vi "VisualizeNetwork.vi"() -> ()   [LabVIEW 2014, in "Visualization.lvlib" / "VisualizeNetwork_class.lvclass"]
uses:
  VisualizeNetwork_class.lvclass
  Framework/Bus_class/Bus.lvclass
  VisializeBase_class/Typedefs/VisualizeData.ctl
  VisializeBase_class/Typedefs/clVisualizeData.ctl
  Modules/EventPlugins/EventPluginBaseClass/TypeDefs/clEvtReportArray.ctl
  Modules/EventPlugins/EventPluginBaseClass/TypeDefs/clEvtReport.ctl
  Modules/EventPlugins/EventPluginBaseClass/TypeDefs/dblEvtSignalArray.ctl
  Modules/NetworkImpairmentModule/PublicAPI/Arguments/Broadcasts/dblNetworkTime.ctl
  Modules/NetworkImpairmentModule/PublicAPI/Arguments/Broadcasts/dblPktLoss.ctl
  Modules/FlagImpairModule/PublicAPI/Arguments/Broadcasts/ui32FlagImpairmentArray.ctl
  Framework/Bus_class/Broadcast/Typedefs/clDidInit.ctl
  QMH/Typedefs/clNetImpairmentTime.ctl
  QMH/Typedefs/clNetIPktLoss.ctl
  QMH/Typedefs/clFlagImpairArray.ctl
  VisializeBase_class/Requests/clUserEventType.ctl
  <vilib>/event_ctls.llb/usereventprio.ctl
  <vilib>/Utility/miscctls.llb/LVStringsAndValuesArrayTypeDef_U8.ctl
  QMH/Typedefs/clEvtRptArray.ctl
  QMH/Typedefs/clPmuImpairRptArray.ctl
  QMH/Typedefs/clEvtRptSignal.ctl
  <vilib>/Utility/error.llb/Error Cluster From Error Code.vi
  <vilib>/ErrorRing/Error Ring.xnode
  VisializeBase_class/VisualizeBase_class.lvclass
  <userlib>/NIST/NISTErrorLib/NISTErrorLib.lvlib
  Framework/Bus_class/Bus_class.lvlib
  Modules/EventModule/EventModule.lvlib
  Modules/PmuImpairModule/PmuImpairModule.lvlib
  Modules/NetworkImpairmentModule/NetworkImpairmentModule.lvlib
  Modules/FlagImpairModule/FlagImpairModule.lvlib
  Modules/EventPlugins/EventPluginBaseClass/EventPluginBaseClass.lvclass
  VisualizeApp_class/VisualizeAppBase_class.lvclass
panel:
  in  "QueName":string="NetQue"
  out "ImpairPlot":cluster{dbl[], i32[]}[](graph) caption="Event Outputs and Impaired Network Outputs Over Time"
  out "Total Network Delay":T1(graph)
  out "Lost Packets":cluster{"NetworkTime":dbl, "BusIndex":u16}[](graph)
  in  "Bus Number":u8(ring) items=["", "1"]
  out "ErrorArray":errorcluster[](array[cluster])
  in  "btnStop":bool
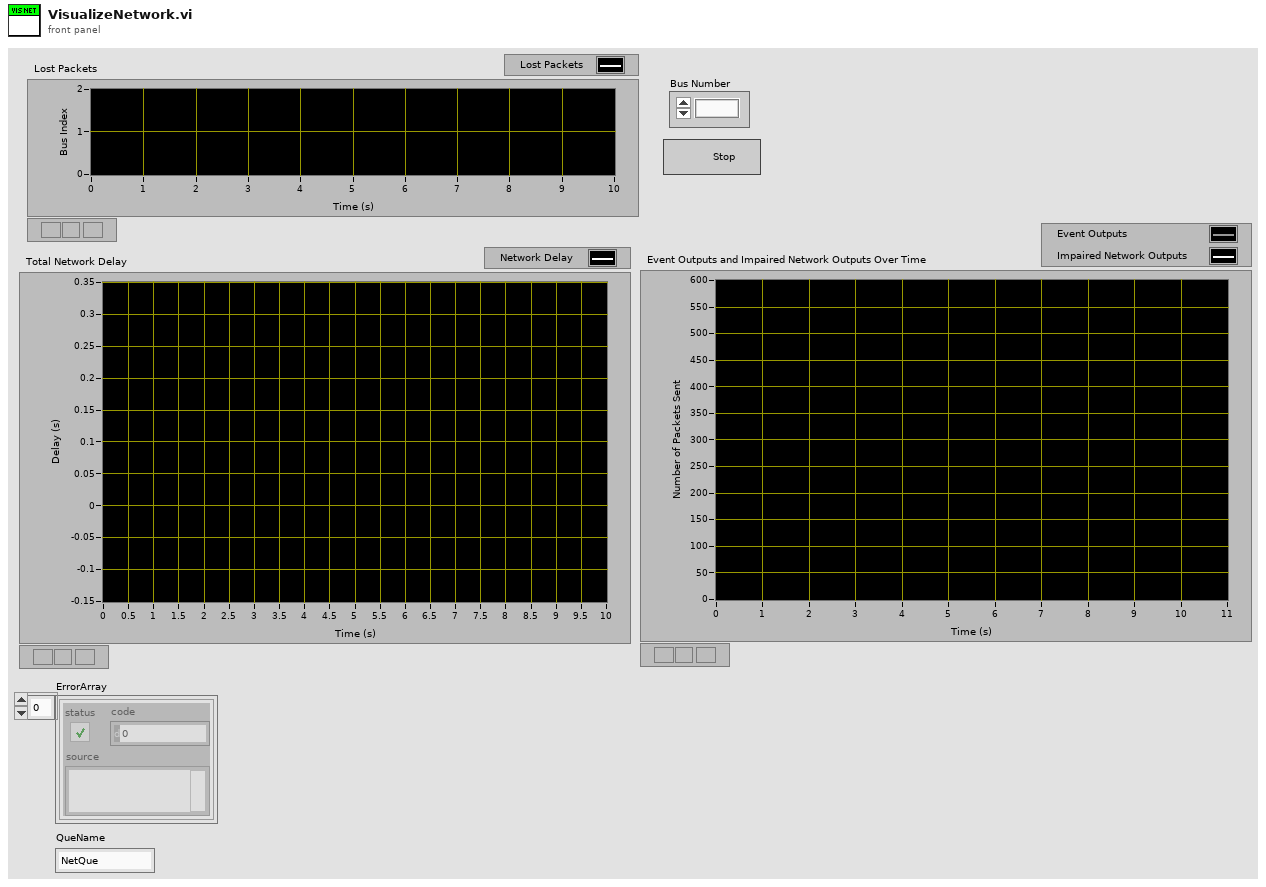
[diagram p1: front panel]
types:
  T1 = cluster{"dblNetworkTime":dbl[], "TimeArray":dbl[]}
  T2 = typedef "Visualization.lvlib/VisualizeBase_class.lvclass/VisualizeData.ctl" = T3[]
  T3 = typedef "Visualization.lvlib/VisualizeAppBase_class.lvclass/clVisualizeData.ctl" = cluster{"clEvtReportArray":T4, "dblEventSignalArray":T6, "clPmuImpairRptArray":T4, "dblNetworkTime":T7, "dblPktLoss":T8, "FlagImpairArray":T9, "TimeArray":dbl[]}
  T4 = typedef "EventPlugins.lvlib/EventPluginBaseClass.lvclass/clEvtReportArray.ctl" = T5[]
  T5 = typedef "EventPlugins.lvlib/EventPluginBaseClass.lvclass/clEvtReport.ctl" = cluster{"Timestamp":dbl, "Synx":cdb[], "Freq":dbl, "ROCOF":dbl, "ID":i16}
  T6 = typedef "EventPlugins.lvlib/EventPluginBaseClass.lvclass/dblEvtSignalArray.ctl" = dbl[][]
  T7 = typedef "NetworkImpairmentModule.lvlib/dblNetworkTime.ctl" = dbl[]
  T8 = typedef "NetworkImpairmentModule.lvlib/dblPktLoss.ctl" = dbl[]
  T9 = typedef "FlagImpairModule.lvlib/ui32FlagImpairmentArray.ctl" = u32[]
  T10 = typedef "Visualization.lvlib/VisualizeBase_class.lvclass/clRequestEvents.ctl" = cluster{"StopRequest":refnum<user-event>}
  T11 = typedef "Bus_class.lvlib/clBroadcastEvents.ctl" = cluster{"DidInit":refnum<user-event>, "DidStop":refnum<user-event>}
  T12 = typedef "EventModule.lvlib/clBroadcastEvents.ctl" = cluster{"DidInit":refnum<user-event>, "StatusUpdate":refnum<user-event>, "ErrorReport":refnum<user-event>, "DidStop":refnum<user-event>, "ReadEvtConfig":refnum<user-event>, "ReadTimeArray":refnum<user-event>, "ReadEvtParams":refnum<user-event>, "GetEvtReportArray":refnum<user-event>, "ReadPathToPlugin":refnum<user-event>, "GetEvtSignal":refnum<user-event>, "ReadBusNumber":refnum<user-event>}
  T13 = typedef "PmuImpairModule.lvlib/clBroadcastEvents.ctl" = cluster{"DidInit":refnum<user-event>, "StatusUpdate":refnum<user-event>, "ErrorReport":refnum<user-event>, "DidStop":refnum<user-event>, "ImpairConfig":refnum<user-event>, "ImpairParams":refnum<user-event>, "ImpairReports":refnum<user-event>, "PathToPlugin":refnum<user-event>, "BusNumber":refnum<user-event>}
  T14 = typedef "NetworkImpairmentModule.lvlib/clBroadcastEvents.ctl" = cluster{"DidInit":refnum<user-event>, "StatusUpdate":refnum<user-event>, "ErrorReport":refnum<user-event>, "DidStop":refnum<user-event>, "ReadNetImpParams":refnum<user-event>, "ReadLossThreshold":refnum<user-event>, "GetNetworkTime":refnum<user-event>, "GetPktLoss":refnum<user-event>, "ReadPathToPlugin":refnum<user-event>}
  T15 = typedef "FlagImpairModule.lvlib/clBroadcastEvents.ctl" = cluster{"DidInit":refnum<user-event>, "StatusUpdate":refnum<user-event>, "ErrorReport":refnum<user-event>, "DidStop":refnum<user-event>, "ReadFlagImpairConfig":refnum<user-event>, "ReadPluginINIFilePath":refnum<user-event>, "ReadFlagImpairParams":refnum<user-event>, "ReadTimeArray":refnum<user-event>, "GetFlagImpairment":refnum<user-event>}
  T16 = cluster{"BusNumberRef":refnum<vi>, "ImpairPlot":refnum<vi>, "Lost Packets":refnum<vi>, "Total Network Delay":refnum<vi>}
  T17 = typedef "LVStringsAndValuesArrayTypeDef_U8.ctl" = cluster{"String":string, "Value":u8}[]
  T18 = typedef "Visualization.lvlib/VisualizeBase_class.lvclass/clEvtRptArray.ctl" = cluster{"BusIndex":i32, "clImpairReportArray":T4}
  T19 = typedef "Visualization.lvlib/VisualizeBase_class.lvclass/clPmuImpairRptArray.ctl" = cluster{"BusIndex":i32, "clImpairReportArray":T4}
  T20 = typedef "Visualization.lvlib/VisualizeBase_class.lvclass/clNetImpairmentTime.ctl" = cluster{"BusIndex":i32, "clNetImpairTimeArray":T7}
  T21 = typedef "Visualization.lvlib/VisualizeBase_class.lvclass/clNetIPktLoss.ctl" = cluster{"BusIndex":i32, "clNetPktLoss":T8}
  T22 = typedef "Visualization.lvlib/VisualizeBase_class.lvclass/clFlagImpairArray.ctl" = cluster{"BusIndex":i32, "FlagImpairArray":T9}
  T23 = typedef "Visualization.lvlib/VisualizeBase_class.lvclass/clEvtRptSignal.ctl" = cluster{"BusIndex":i32, "dblEventSignalArray":T6}
  T24 = typedef "Visualization.lvlib/VisualizeBase_class.lvclass/clUserEventType.ctl" = cluster{"BusIndex":i8, "Data":variant}
  T25 = typedef "usereventprio.ctl" = enum32{"high priority", "normal priority"}
  T26 = typedef "Bus_class.lvlib/clDidInit.ctl" = cluster{"Bus":refnum<vi>, "Init?":bool}
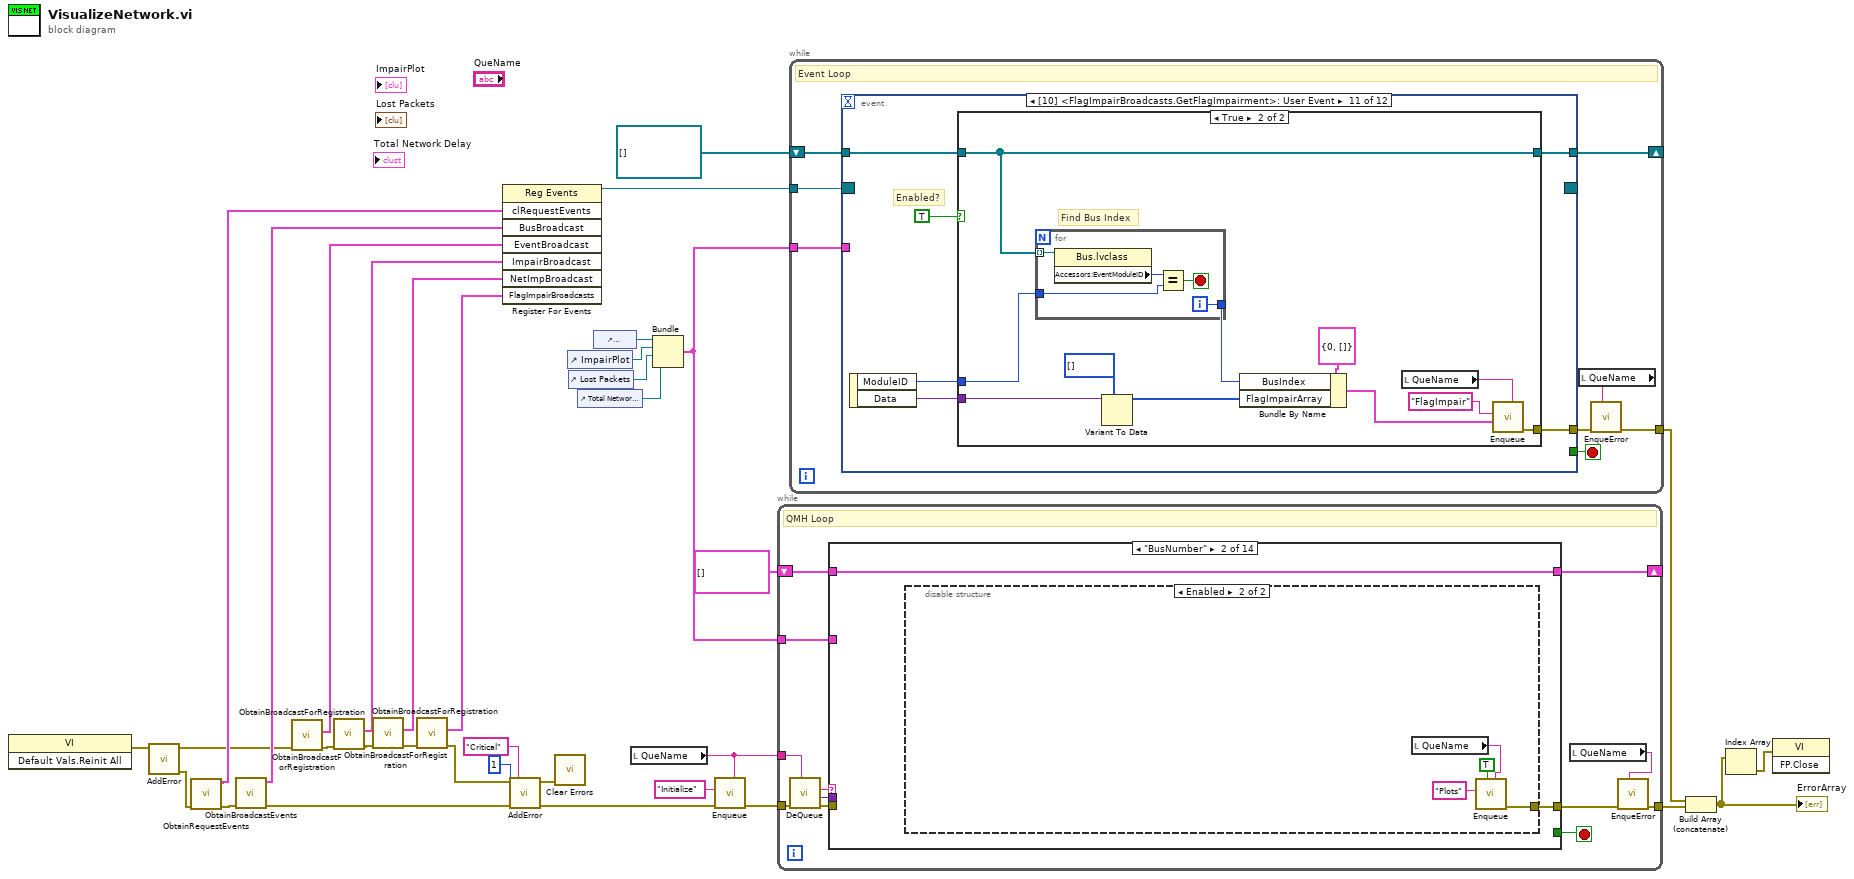
[diagram p0: block diagram]
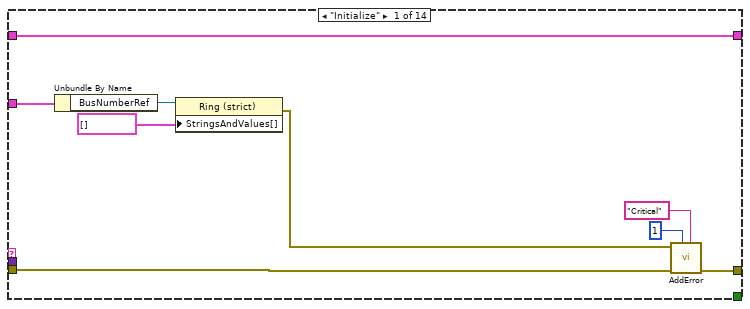
[diagram p2: hidden frame]
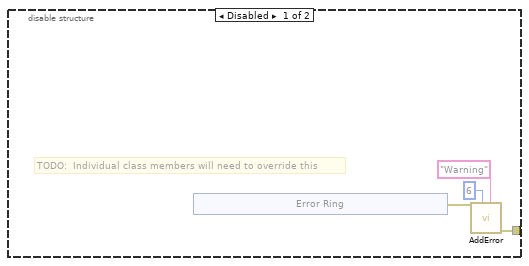
[diagram p3: hidden frame]
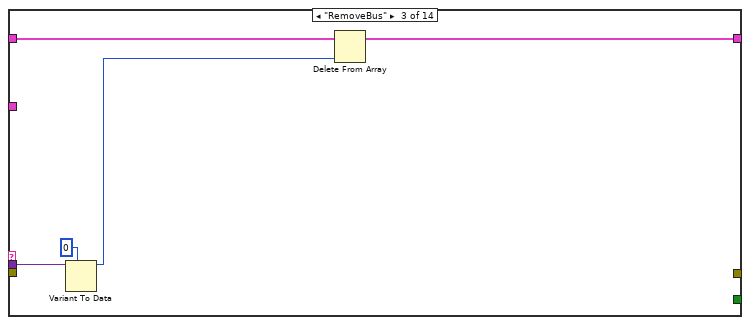
[diagram p4: hidden frame]
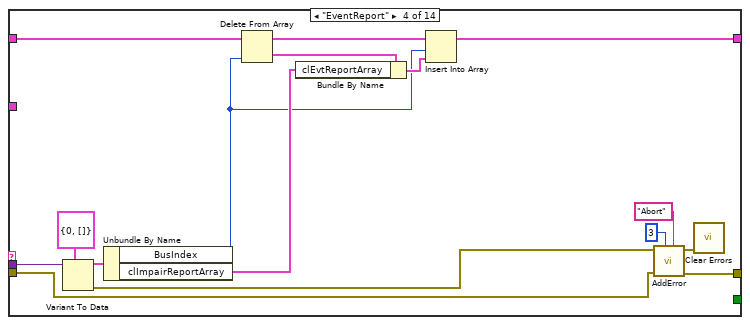
[diagram p5: hidden frame]
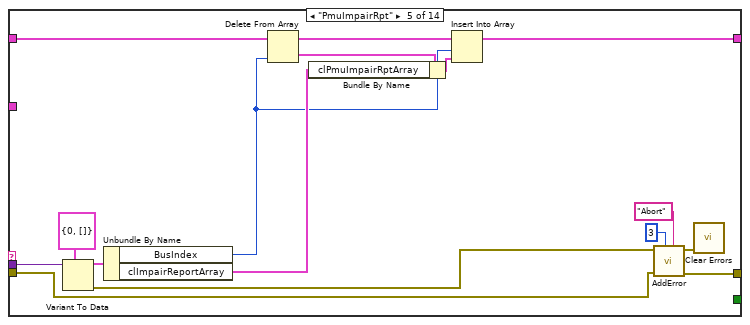
[diagram p6: hidden frame]
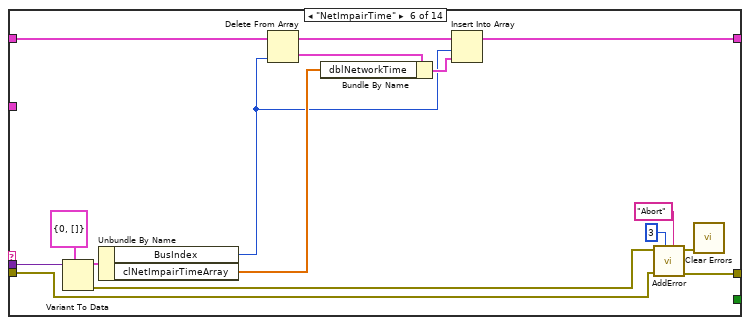
[diagram p7: hidden frame]
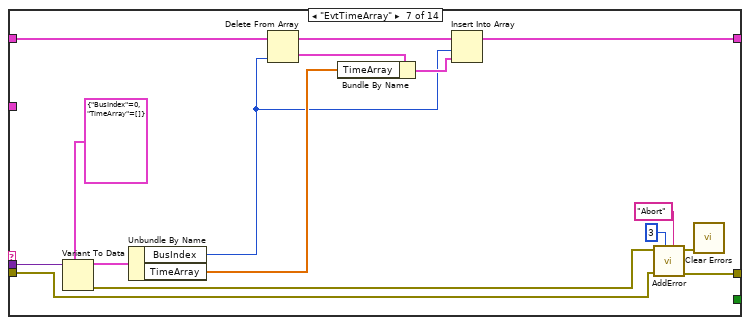
[diagram p8: hidden frame]
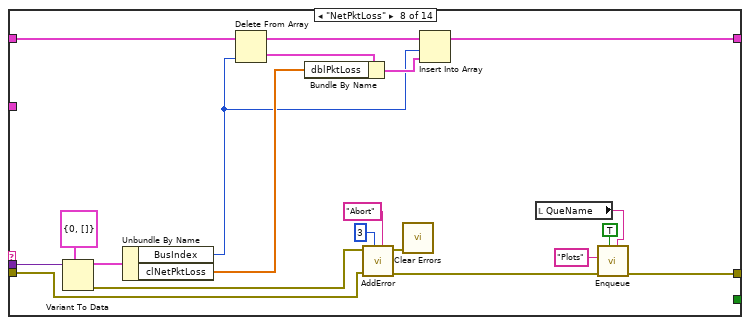
[diagram p9: hidden frame]
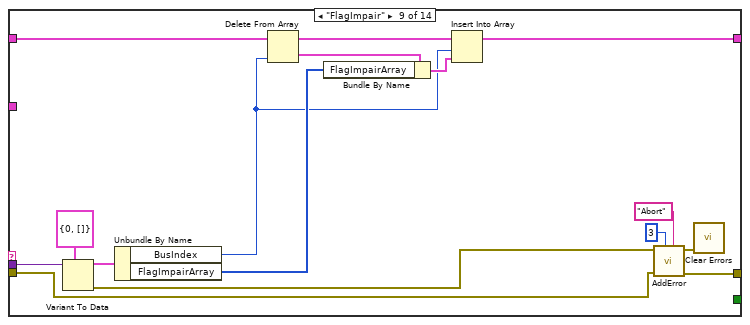
[diagram p10: hidden frame]
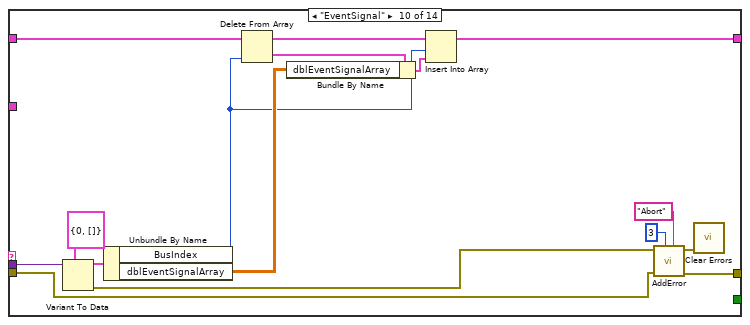
[diagram p11: hidden frame]
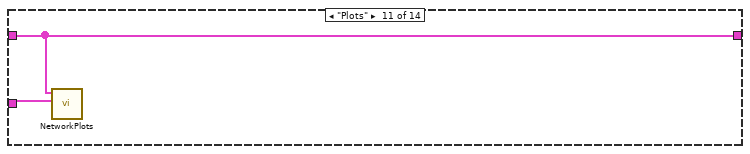
[diagram p12: hidden frame]
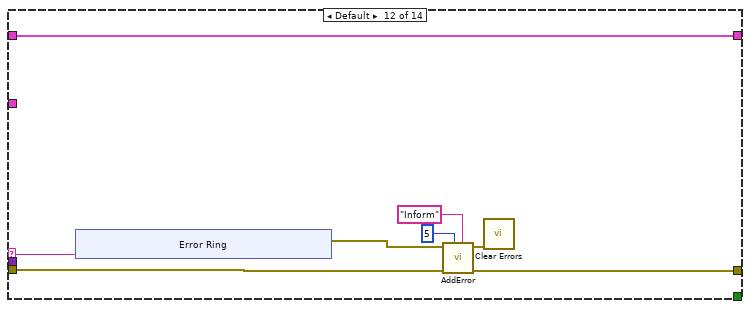
[diagram p13: hidden frame]
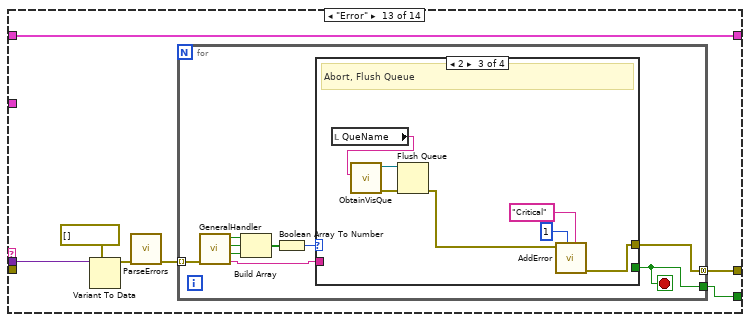
[diagram p14: hidden frame]
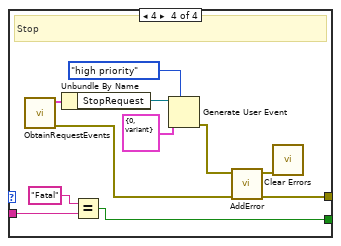
[diagram p17: hidden frame]
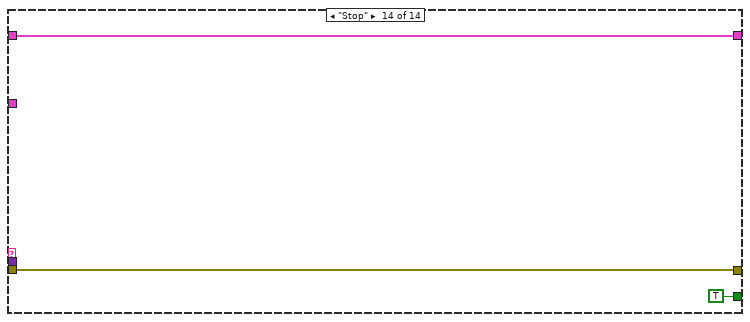
[diagram p18: hidden frame]
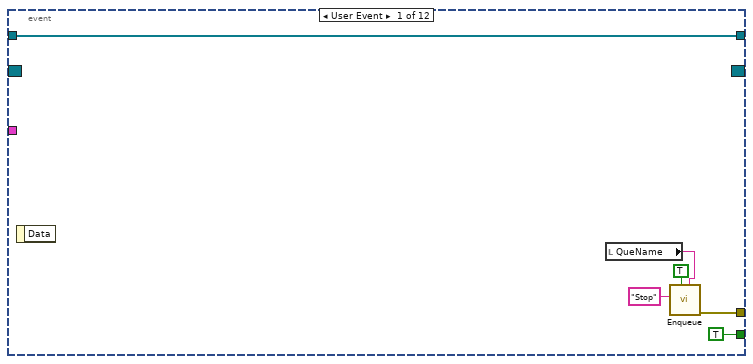
[diagram p19: hidden frame]
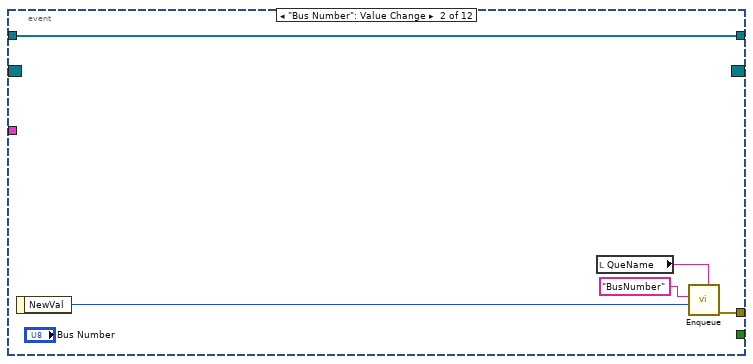
[diagram p20: hidden frame]
diagram:
  n1 = invoke class="VI" method="Default Vals.Reinit All"() -> (error out=w24:errorcluster)  [unwired: 3 in, 2 out]
  n2 = call <userlib>:"AddError.vi"("error in (no error)"=w24) -> ("ErrorArray"=w23:errorcluster[], "error out"=w15:errorcluster)  [unwired: 9 in]
  n3 = call "ObtainRequestEvents.vi"("Error"=w23) -> ("Error"=w28:errorcluster[], "clRequestEvents"=w32:T10)  [unwired: 9 in]
  n4 = call "ObtainBroadcastEvents.vi"("ErrorArray"=w28) -> ("ErrorArray"=w14:errorcluster[], "BusBroadcast"=w27:T11)  [unwired: 9 in]
  n5 = call "ObtainBroadcastForRegistration.vi"("error in (no error)"=w15) -> ("error out"=w18:errorcluster, "EventBroadcast"=w22:T12)  [unwired: 9 in]
  n6 = call "ObtainBroadcastForRegistration.vi"("error in (no error)"=w18) -> ("error out"=w17:errorcluster, "ImpairBroadcast"=w21:T13)  [unwired: 9 in]
  n7 = call "ObtainBroadcastForRegistration.vi"("error in (no error)"=w17) -> ("error out"=w16:errorcluster, "NetImpBroadcast"=w20:T14)  [unwired: 9 in]
  n8 = call "ObtainBroadcastForRegistration.vi"("error in (no error)"=w16) -> ("error out"=w13:errorcluster, "FlagImpairBroadcasts"=w19:T15)  [unwired: 9 in]
  n9 = register-events(w32, w27, w22, w21, w20, w19) -> (reference out=w31:refnum<event-registration>)  [unwired: 2 in, 1 out]
  n10 = call <userlib>:"AddError.vi"("Severity"="Critical" ("String"), "Priority"=u8 1, "ErrorArray"=w14, "error in (no error)"=w13) -> ("ErrorArray"=w10:errorcluster[], "error out"=w7:errorcluster)  [unwired: 6 in]
  n11 = call <vilib>:"Clear Errors.vi"("error in (no error)"=w7) -> ()  [unwired: 5 in, 2 out]
  n12 = control-ref of="ImpairPlot"() -> (w4:refnum<vi>)
  n13 = control-ref of="Lost Packets"() -> (w6:refnum<vi>)
  n14 = control-ref of="Total Network Delay"() -> (w5:refnum<vi>)
  n15 = control-ref of="BusNumberRef"() -> (w26:refnum<vi>)
  n16 = local read "QueName"() -> (w3:string)
  n17 = Bundle("BusNumberRef"=w26, "ImpairPlot"=w4, "Lost Packets"=w6, "Total Network Delay"=w5) -> (w8:T16)  [unwired: 1 in]
  n18 = call "Enqueue.vi"("QueName"=w3, "Error"=w10, "Message"="Initialize") -> ("Error"=w33:errorcluster[])  [unwired: 8 in]
  n19 = while {
    tunnel: w33 -> [w46]
    tunnel: [w40] -> w30
    tunnel: w8 -> [w39]
    shift-right: [w37] -> _
    shift-left: T2 [] ("VisualizeData") -> [w38]
    tunnel: w3 -> [w36]
    stop <- w41 stop-if-true
    # "QMH Loop"
    n20 = call "DeQueue.vi"("QueName"=w36, "Error"=w46) -> ("Error"=w43:errorcluster[], "Data"=w44:variant, "Message"=w45:string)  [unwired: 7 in]
    n21 = case shown="\"BusNumber\"" w45 {
      selector: w45 -> [_ _ _ _ _ _ _ _ _ _ _ w201 _ _]
      tunnel: w44 -> [_ _ w75 w91 w107 w123 w139 w159 w175 w191 _ _ w215 _]
      tunnel: w43 -> [w52 _ _ w76 w92 w108 w125 w145 w160 w176 _ w199 _ w244]
      tunnel: [w51 w57 _ w81 w97 w113 w130 w143 w165 w181 _ w198 w211 w244] -> w42
      tunnel: [_ _ _ _ _ _ _ _ _ _ _ _ w210 TRUE] -> w41
      tunnel: w39 -> [w55 _ _ _ _ _ _ _ _ _ w192 _ _ _]
      tunnel: w38 -> [w47 w56 w73 w87 w103 w119 w136 w155 w171 w187 w193 w194 w209 w243]
      tunnel: [w47 w56 w72 w88 w104 w120 w137 w156 w172 w188 w193 w194 w209 w243] -> w37
      frame "Initialize" {
        n22 = Unbundle By Name(w55) -> ("BusNumberRef"=w54:refnum<vi>)
        n23 = property class="Ring (strict)"(reference=w54, "StringsAndValues[]"=T17 [] ("Strings And Values []")) -> (error out=w50:errorcluster)  [unwired: 1 in, 1 out]
        n24 = call <userlib>:"AddError.vi"("Severity"="Critical" ("String"), "Priority"=u8 1, "ErrorArray"=w52, "error in (no error)"=w50) -> ("ErrorArray"=w51:errorcluster[])  [unwired: 6 in, 1 out]
      }
      frame "BusNumber" {
        n25 = disable-structure shown="Enabled" {
          disable-tunnel: [w61 w67] -> w57
          frame Disabled {
            # "TODO:  Individual class members will need to override this"
            n26 = xnode "Error Ring"() -> ("error out"=w60:errorcluster)
            n27 = call <userlib>:"AddError.vi"("Severity"="Warning" ("String"), "Priority"=u8 6, "error in (no error)"=w60) -> ("ErrorArray"=w61:errorcluster[])  [unwired: 7 in, 1 out]
          }
          frame Enabled {
            n28 = local read "QueName"() -> (w70:string)
            n29 = call "Enqueue.vi"("QueName"=w70, "Priority? (F)"=TRUE, "Message"="Plots") -> ("Error"=w67:errorcluster[])  [unwired: 8 in]
          }
        }
      }
      frame "RemoveBus" {
        n30 = Variant To Data(type=0, Variant=w75) -> (data=w71:i32)  [unwired: 1 in, 1 out]
        n31 = Delete From Array(array=w73, index=w71) -> (array with subset deleted=w72:T2)  [unwired: 1 in, 1 out]
      }
      frame "EventReport" {
        n32 = Variant To Data(type=T18 {"BusIndex"=0, "clImpairReportArray"=[]} ("clEvtReportArray"), Variant=w91) -> (data=w89:T18, error out=w80:errorcluster)  [unwired: 1 in]
        n33 = Unbundle By Name(w89) -> ("BusIndex"=w82:i32, "clImpairReportArray"=w84:T4)
        n34 = Delete From Array(array=w87, index=w82) -> (deleted portion=w85:T3, array with subset deleted=w86:T2)  [unwired: 1 in]
        n35 = Bundle By Name(cluster=w85, "clEvtReportArray"=w84) -> (w83:T3)
        n36 = Insert Into Array(array=w86, index=w82, new element=w83) -> (w88:T2)
        n37 = call <userlib>:"AddError.vi"("Severity"="Abort" ("String"), "Priority"=u8 3, "ErrorArray"=w76, "error in (no error)"=w80) -> ("ErrorArray"=w81:errorcluster[], "error out"=w79:errorcluster)  [unwired: 6 in]
        n38 = call <vilib>:"Clear Errors.vi"("error in (no error)"=w79) -> ()  [unwired: 5 in, 2 out]
      }
      frame "PmuImpairRpt" {
        n39 = Variant To Data(type=T19 {"BusIndex"=0, "clImpairReportArray"=[]} ("clImpairReportArray"), Variant=w107) -> (data=w105:T19, error out=w96:errorcluster)  [unwired: 1 in]
        n40 = Unbundle By Name(w105) -> ("BusIndex"=w98:i32, "clImpairReportArray"=w100:T4)
        n41 = Delete From Array(array=w103, index=w98) -> (deleted portion=w101:T3, array with subset deleted=w102:T2)  [unwired: 1 in]
        n42 = Bundle By Name(cluster=w101, "clPmuImpairRptArray"=w100) -> (w99:T3)
        n43 = Insert Into Array(array=w102, index=w98, new element=w99) -> (w104:T2)
        n44 = call <userlib>:"AddError.vi"("Severity"="Abort" ("String"), "Priority"=u8 3, "ErrorArray"=w92, "error in (no error)"=w96) -> ("ErrorArray"=w97:errorcluster[], "error out"=w95:errorcluster)  [unwired: 6 in]
        n45 = call <vilib>:"Clear Errors.vi"("error in (no error)"=w95) -> ()  [unwired: 5 in, 2 out]
      }
      frame "NetImpairTime" {
        n46 = Variant To Data(type=T20 {"BusIndex"=0, "clNetImpairTimeArray"=[]} ("clImpairReportArray"), Variant=w123) -> (data=w121:T20, error out=w112:errorcluster)  [unwired: 1 in]
        n47 = Unbundle By Name(w121) -> ("BusIndex"=w114:i32, "clNetImpairTimeArray"=w116:T7)
        n48 = Delete From Array(array=w119, index=w114) -> (deleted portion=w117:T3, array with subset deleted=w118:T2)  [unwired: 1 in]
        n49 = Bundle By Name(cluster=w117, "dblNetworkTime"=w116) -> (w115:T3)
        n50 = Insert Into Array(array=w118, index=w114, new element=w115) -> (w120:T2)
        n51 = call <userlib>:"AddError.vi"("Severity"="Abort" ("String"), "Priority"=u8 3, "ErrorArray"=w108, "error in (no error)"=w112) -> ("ErrorArray"=w113:errorcluster[], "error out"=w111:errorcluster)  [unwired: 6 in]
        n52 = call <vilib>:"Clear Errors.vi"("error in (no error)"=w111) -> ()  [unwired: 5 in, 2 out]
      }
      frame "EvtTimeArray" {
        n53 = Variant To Data(type=cluster{"BusIndex":i32, "TimeArray":dbl[]} {"BusIndex"=0, "TimeArray"=[]} ("cluster"), Variant=w139) -> (data=w138:cluster{"BusIndex":i32, "TimeArray":dbl[]}, error out=w129:errorcluster)  [unwired: 1 in]
        n54 = Unbundle By Name(w138) -> ("BusIndex"=w131:i32, "TimeArray"=w133:dbl[])
        n55 = Delete From Array(array=w136, index=w131) -> (deleted portion=w134:T3, array with subset deleted=w135:T2)  [unwired: 1 in]
        n56 = Bundle By Name(cluster=w134, "TimeArray"=w133) -> (w132:T3)
        n57 = Insert Into Array(array=w135, index=w131, new element=w132) -> (w137:T2)
        n58 = call <userlib>:"AddError.vi"("Severity"="Abort" ("String"), "Priority"=u8 3, "ErrorArray"=w125, "error in (no error)"=w129) -> ("ErrorArray"=w130:errorcluster[], "error out"=w128:errorcluster)  [unwired: 6 in]
        n59 = call <vilib>:"Clear Errors.vi"("error in (no error)"=w128) -> ()  [unwired: 5 in, 2 out]
      }
      frame "NetPktLoss" {
        n60 = Variant To Data(type=T21 {"BusIndex"=0, "clNetPktLoss"=[]} ("clNetPktLoss"), Variant=w159) -> (data=w157:T21, error out=w149:errorcluster)  [unwired: 1 in]
        n61 = Unbundle By Name(w157) -> ("BusIndex"=w150:i32, "clNetPktLoss"=w152:T8)
        n62 = Delete From Array(array=w155, index=w150) -> (deleted portion=w153:T3, array with subset deleted=w154:T2)  [unwired: 1 in]
        n63 = Bundle By Name(cluster=w153, "dblPktLoss"=w152) -> (w151:T3)
        n64 = call <userlib>:"AddError.vi"("Severity"="Abort" ("String"), "Priority"=u8 3, "ErrorArray"=w145, "error in (no error)"=w149) -> ("ErrorArray"=w144:errorcluster[], "error out"=w148:errorcluster)  [unwired: 6 in]
        n65 = call <vilib>:"Clear Errors.vi"("error in (no error)"=w148) -> ()  [unwired: 5 in, 2 out]
        n66 = Insert Into Array(array=w154, index=w150, new element=w151) -> (w156:T2)
        n67 = local read "QueName"() -> (w140:string)
        n68 = call "Enqueue.vi"("QueName"=w140, "Priority? (F)"=TRUE, "Error"=w144, "Message"="Plots") -> ("Error"=w143:errorcluster[])  [unwired: 7 in]
      }
      frame "FlagImpair" {
        n69 = Variant To Data(type=T22 {"BusIndex"=0, "FlagImpairArray"=[]} ("clFlagImpairArray"), Variant=w175) -> (data=w173:T22, error out=w164:errorcluster)  [unwired: 1 in]
        n70 = Unbundle By Name(w173) -> ("BusIndex"=w166:i32, "FlagImpairArray"=w168:T9)
        n71 = Delete From Array(array=w171, index=w166) -> (deleted portion=w169:T3, array with subset deleted=w170:T2)  [unwired: 1 in]
        n72 = Bundle By Name(cluster=w169, "FlagImpairArray"=w168) -> (w167:T3)
        n73 = Insert Into Array(array=w170, index=w166, new element=w167) -> (w172:T2)
        n74 = call <userlib>:"AddError.vi"("Severity"="Abort" ("String"), "Priority"=u8 3, "ErrorArray"=w160, "error in (no error)"=w164) -> ("ErrorArray"=w165:errorcluster[], "error out"=w163:errorcluster)  [unwired: 6 in]
        n75 = call <vilib>:"Clear Errors.vi"("error in (no error)"=w163) -> ()  [unwired: 5 in, 2 out]
      }
      frame "EventSignal" {
        n76 = Variant To Data(type=T23 {"BusIndex"=0, "dblEventSignalArray"=[]} ("clEvtReportArray"), Variant=w191) -> (data=w189:T23, error out=w180:errorcluster)  [unwired: 1 in]
        n77 = Unbundle By Name(w189) -> ("BusIndex"=w182:i32, "dblEventSignalArray"=w184:T6)
        n78 = Delete From Array(array=w187, index=w182) -> (deleted portion=w185:T3, array with subset deleted=w186:T2)  [unwired: 1 in]
        n79 = Bundle By Name(cluster=w185, "dblEventSignalArray"=w184) -> (w183:T3)
        n80 = Insert Into Array(array=w186, index=w182, new element=w183) -> (w188:T2)
        n81 = call <userlib>:"AddError.vi"("Severity"="Abort" ("String"), "Priority"=u8 3, "ErrorArray"=w176, "error in (no error)"=w180) -> ("ErrorArray"=w181:errorcluster[], "error out"=w179:errorcluster)  [unwired: 6 in]
        n82 = call <vilib>:"Clear Errors.vi"("error in (no error)"=w179) -> ()  [unwired: 5 in, 2 out]
      }
      frame "Plots" {
        n83 = call "NetworkPlots.vi"("ControlRefs"=w192, "VisualizeData"=w193) -> ()  [unwired: 10 in]
      }
      frame Default {
        n84 = xnode "Error Ring"("parameter 0"=w201) -> ("error out"=w200:errorcluster)
        n85 = call <userlib>:"AddError.vi"("Severity"="Inform" ("String"), "Priority"=u8 5, "ErrorArray"=w199, "error in (no error)"=w200) -> ("ErrorArray"=w198:errorcluster[], "error out"=w197:errorcluster)  [unwired: 6 in]
        n86 = call <vilib>:"Clear Errors.vi"("error in (no error)"=w197) -> ()  [unwired: 5 in, 2 out]
      }
      frame "Error" {
        n87 = Variant To Data(type=errorcluster[] [], Variant=w215) -> (data=w213:errorcluster[])  [unwired: 1 in, 1 out]
        n88 = call <userlib>:"ParseErrors.vi"("ErrorArray"=w213) -> ("ErrorArray"=w212:errorcluster[])  [unwired: 8 in, 2 out]
        n89 = for {
          tunnel: w212 -> [w224] mode=indexing
          tunnel: [w218] -> w211 mode=concatenating
          tunnel: [w216] -> w210
          stop <- w216 stop-if-true
          n90 = call <userlib>:"GeneralHandler.vi"("error in (no error)"=w224) -> ("Severity"=w217:string, "Stop"=w221:bool, "Abort"=w222:bool, "Continue"=w223:bool)  [unwired: 7 in]
          n91 = Build Array(w223, w222, w221) -> (w220:bool[])
          n92 = Boolean Array To Number(Boolean array=w220) -> (number=w219:u32)
          n93 = case shown="2" w219 {
            tunnel: [_ _ w229 w240] -> w218
            tunnel: w217 -> [_ _ _ w234]
            tunnel: [_ _ _ w232] -> w216
            frame 0, Default {
              # "No Dialog"
            }
            frame 1 {
              # "Continue"
            }
            frame 2 {
              # "Abort, Flush Queue"
              n94 = local read "QueName"() -> (w225:string)
              n95 = call "ObtainVisQue.vi"("QueName"=w225) -> ("error out"=w231:errorcluster, "queue out"=w230:refnum<queue>)  [unwired: 9 in]
              n96 = Flush Queue(queue=w230, error in (no error)=w231) -> (error out=w228:errorcluster)  [unwired: 2 out]
              n97 = call <userlib>:"AddError.vi"("Severity"="Critical" ("String"), "Priority"=u8 1, "error in (no error)"=w228) -> ("ErrorArray"=w229:errorcluster[])  [unwired: 7 in, 1 out]
            }
            frame 4 {
              # "Stop"
              n98 = call "ObtainRequestEvents.vi"() -> ("Error"=w238:errorcluster[], "clRequestEvents"=w242:T10)  [unwired: 10 in]
              n99 = Unbundle By Name(w242) -> ("StopRequest"=w241:refnum<user-event>)
              n100 = Equal?(x="Fatal", y=w234) -> (x = y?=w232:bool)
              n101 = Generate User Event(priority (normal)=usereventprio."high priority", user event=w241, event data cluster=T24 {"BusIndex"=0, "Data"=variant} ("event data")) -> (error out=w239:errorcluster)  [unwired: 1 in, 1 out]
              n102 = call <userlib>:"AddError.vi"("ErrorArray"=w238, "error in (no error)"=w239) -> ("ErrorArray"=w240:errorcluster[], "error out"=w235:errorcluster)  [unwired: 8 in]
              n103 = call <vilib>:"Clear Errors.vi"("error in (no error)"=w235) -> ()  [unwired: 5 in, 2 out]
            }
          }
        }
      }
      frame "Stop" {
      }
    }
    n104 = local read "QueName"() -> (w35:string)
    n105 = call "EnqueError.vi"("QueName"=w35, "Error"=w42) -> ("Error"=w40:errorcluster[])  [unwired: 9 in]
  }
  n106 = while {
    tunnel: w31 -> [w253]
    tunnel: [w250] -> w29
    tunnel: w8 -> [w249]
    shift-right: [w247] -> _
    shift-left: refnum<class "Bus.lvclass">[] [] -> [w248]
    stop <- w252 stop-if-true
    # "Event Loop"
    n107 = event shown="[10] <FlagImpairBroadcasts.GetFlagImpairment>: User Event" {
      selector: w253 -> [_ _ _ _ _ _ _ _ _ _ _ _]
      dyn-events: [_ _ w273 _ _ _ _ _ _ _ _ _] -> _
      timeout: _ -> [_ _ _ _ _ _ _ _ _ _ _ _]
      tunnel: [TRUE _ _ _ _ _ _ _ _ _ _ _] -> w252
      tunnel: [w258 w264 w276 w294 w299 w329 w352 w375 w398 w421 w444 w471] -> w251
      tunnel: w249 -> [_ _ w286 w298 _ _ _ _ _ _ _ _]
      tunnel: w248 -> [w255 w261 w285 w297 w303 w332 w355 w378 w401 w424 w447 w465]
      tunnel: [w255 w261 w282 w296 w302 w327 w350 w373 w396 w419 w442 w465] -> w247
      event User Event {
        n108 = event-data() -> ()  [unwired: 1 in, 1 out]
        n109 = local read "QueName"() -> (w254:string)
        n110 = call "Enqueue.vi"("QueName"=w254, "Priority? (F)"=TRUE, "Message"="Stop") -> ("Error"=w258:errorcluster[])  [unwired: 8 in]
      }
      event "Bus Number": Value Change {
        n111 = event-data() -> ("NewVal"=w263:u8)  [unwired: 1 in]
        n112 = local read "QueName"() -> (w260:string)
        n113 = call "Enqueue.vi"("QueName"=w260, "Data"=w263, "Message"="BusNumber") -> ("Error"=w264:errorcluster[])  [unwired: 8 in]
      }
      event User Event {
        n114 = event-data() -> ("Data"=w289:variant)  [unwired: 1 in]
        n115 = Unbundle By Name(w286) -> ("BusNumberRef"=w284:refnum<vi>)
        n116 = Variant To Data(type=T26 {"Bus"=refnum, "Init?"=FALSE} ("clBusDidInit"), Variant=w289) -> (data=w287:T26)  [unwired: 1 in, 1 out]
        n117 = Unbundle By Name(w287) -> ("Bus"=w283:refnum<vi>)
        n118 = call "AddBus.vi"("BusRef"=w283, "BusNumberRef"=w284, "BusArray"=w285) -> ("BusArray"=w282:refnum<class "Bus.lvclass">[])  [unwired: 8 in]
        n119 = call "ObtainRequestEvents.vi"() -> ("Error"=w268:errorcluster[], "clRequestEvents"=w266:T10)  [unwired: 10 in]
        n120 = call "ObtainBroadcastEvents.vi"("ErrorArray"=w268) -> ("ErrorArray"=w267:errorcluster[], "BusBroadcast"=w265:T11)  [unwired: 9 in]
        n121 = call "ObtainBroadcastForRegistration.vi"() -> ("error out"=w281:errorcluster, "EventBroadcast"=w272:T12)  [unwired: 10 in]
        n122 = call "ObtainBroadcastForRegistration.vi"("error in (no error)"=w281) -> ("error out"=w280:errorcluster, "ImpairBroadcast"=w271:T13)  [unwired: 9 in]
        n123 = call "ObtainBroadcastForRegistration.vi"("error in (no error)"=w280) -> ("error out"=w279:errorcluster, "NetImpBroadcast"=w270:T14)  [unwired: 9 in]
        n124 = call "ObtainBroadcastForRegistration.vi"("error in (no error)"=w279) -> ("error out"=w274:errorcluster, "FlagImpairBroadcasts"=w269:T15)  [unwired: 9 in]
        n125 = register-events(w266, w265, w272, w271, w270, w269) -> (reference out=w273:refnum<event-registration>)  [unwired: 2 in, 1 out]
        n126 = call <userlib>:"AddError.vi"("Severity"="Critical" ("String"), "Priority"=u8 1, "ErrorArray"=w267, "error in (no error)"=w274) -> ("ErrorArray"=w276:errorcluster[], "error out"=w275:errorcluster)  [unwired: 6 in]
        n127 = call <vilib>:"Clear Errors.vi"("error in (no error)"=w275) -> ()  [unwired: 5 in, 2 out]
      }
      event User Event {
        n128 = event-data() -> ("BusNumber"=w291:i8)  [unwired: 1 in]
        n129 = Unbundle By Name(w298) -> ("BusNumberRef"=w295:refnum<vi>)
        n130 = call "RemoveBus.vi"("BusArray"=w297, "BusNumberRef"=w295, "BusNumber"=w291) -> ("BusArray"=w296:refnum<class "Bus.lvclass">[], "BusIndex"=w293:i32)  [unwired: 6 in]
        n131 = local read "QueName"() -> (w290:string)
        n132 = call "Enqueue.vi"("QueName"=w290, "Data"=w293, "Message"="RemoveBus") -> ("Error"=w294:errorcluster[])  [unwired: 8 in]
      }
      event User Event {
        w304 = TRUE  # Enabled?
        n133 = event-data() -> ("ModuleID"=w301:i32, "Data"=w300:variant)  [unwired: 1 in]
        n134 = case shown="True" w304 {
          tunnel: [w305 w321] -> w302
          tunnel: w303 -> [w305 w321]
          tunnel: w301 -> [_ w318]
          tunnel: w300 -> [_ w320]
          tunnel: [_ w308] -> w299
          frame False {
          }
          frame True {
            n135 = Variant To Data(type=dbl[] [], Variant=w320) -> (data=w317:dbl[], error out=w313:errorcluster)  [unwired: 1 in]
            n136 = for {
              tunnel: w321 -> [w326] mode=indexing
              tunnel: w318 -> [w324]
              tunnel: [w322] -> w307
              i -> [w322]
              stop <- w323 stop-if-true
              # "Find Bus Index"
              n137 = property class="Bus.lvclass"(reference=w326) -> ("Accessors:EventModuleID"=w325:i32)  [unwired: 1 in, 2 out]
              n138 = Equal?(x=w325, y=w324) -> (x = y?=w323:bool)
            }
            n139 = call <userlib>:"AddError.vi"("Severity"="Critical" ("String"), "Priority"=u8 1, "error in (no error)"=w313) -> ("ErrorArray"=w309:errorcluster[], "error out"=w312:errorcluster)  [unwired: 7 in]
            n140 = call <vilib>:"Clear Errors.vi"("error in (no error)"=w312) -> ()  [unwired: 5 in, 2 out]
            n141 = Bundle(w307, w317) -> (w316:cluster{i32, dbl[]})  [unwired: 1 in]
            n142 = To Variant(anything=w316) -> (Variant=w315:variant)
            n143 = local read "QueName"() -> (w306:string)
            n144 = call "Enqueue.vi"("QueName"=w306, "Error"=w309, "Data"=w315, "Message"="EvtTimeArray") -> ("Error"=w308:errorcluster[])  [unwired: 7 in]
          }
        }
      }
      event User Event {
        # "Enabled?"
        n145 = event-data() -> ("ModuleID"=w331:i32, "Data"=w330:variant)  [unwired: 1 in]
        n146 = case shown="True" FALSE {
          tunnel: w332 -> [w333 w335]
          tunnel: w331 -> [_ w344]
          tunnel: w330 -> [_ w342]
          tunnel: [_ w339] -> w329
          tunnel: [w333 w335] -> w327
          frame False {
          }
          frame True {
            # "Find Bus Index"
            n147 = for {
              tunnel: w335 -> [w349] mode=indexing
              tunnel: w344 -> [w347]
              tunnel: [w345] -> w343
              i -> [w345]
              stop <- w346 stop-if-true
              n148 = property class="Bus.lvclass"(reference=w349) -> ("Accessors:EventModuleID"=w348:i32)  [unwired: 1 in, 2 out]
              n149 = Equal?(x=w348, y=w347) -> (x = y?=w346:bool)
            }
            n150 = Variant To Data(type=T4 [] ("clEvtReportArray"), Variant=w342) -> (data=w340:T4)  [unwired: 1 in, 1 out]
            n151 = Bundle By Name(cluster=T18 {"BusIndex"=0, "clImpairReportArray"=[]} ("clEvtReportArray"), "BusIndex"=w343, "clImpairReportArray"=w340) -> (w338:T18)
            n152 = local read "QueName"() -> (w334:string)
            n153 = call "Enqueue.vi"("QueName"=w334, "Data"=w338, "Message"="EventReport") -> ("Error"=w339:errorcluster[])  [unwired: 8 in]
          }
        }
      }
      event User Event {
        # "Enabled?"
        n154 = event-data() -> ("ModuleID"=w354:i32, "Data"=w353:variant)  [unwired: 1 in]
        n155 = case shown="True" FALSE {
          tunnel: w355 -> [w356 w358]
          tunnel: w354 -> [_ w367]
          tunnel: w353 -> [_ w365]
          tunnel: [_ w362] -> w352
          tunnel: [w356 w358] -> w350
          frame False {
          }
          frame True {
            # "Find Bus Index"
            n156 = for {
              tunnel: w358 -> [w372] mode=indexing
              tunnel: w367 -> [w370]
              tunnel: [w368] -> w366
              i -> [w368]
              stop <- w369 stop-if-true
              n157 = property class="Bus.lvclass"(reference=w372) -> ("Accessors:EventModuleID"=w371:i32)  [unwired: 1 in, 2 out]
              n158 = Equal?(x=w371, y=w370) -> (x = y?=w369:bool)
            }
            n159 = Variant To Data(type=T6 [] ("dblEventSignalArray"), Variant=w365) -> (data=w363:T6)  [unwired: 1 in, 1 out]
            n160 = Bundle By Name(cluster=T23 {"BusIndex"=0, "dblEventSignalArray"=[]} ("clEvtReportArray"), "BusIndex"=w366, "dblEventSignalArray"=w363) -> (w361:T23)
            n161 = local read "QueName"() -> (w357:string)
            n162 = call "Enqueue.vi"("QueName"=w357, "Data"=w361, "Message"="EventSignal") -> ("Error"=w362:errorcluster[])  [unwired: 8 in]
          }
        }
      }
      event User Event {
        # "Enabled?"
        n163 = event-data() -> ("ModuleID"=w377:i32, "Data"=w376:variant)  [unwired: 1 in]
        n164 = case shown="True" FALSE {
          tunnel: w378 -> [w379 w381]
          tunnel: w377 -> [_ w390]
          tunnel: w376 -> [_ w388]
          tunnel: [_ w385] -> w375
          tunnel: [w379 w381] -> w373
          frame False {
          }
          frame True {
            # "Find Bus Index"
            n165 = for {
              tunnel: w381 -> [w395] mode=indexing
              tunnel: w390 -> [w393]
              tunnel: [w391] -> w389
              i -> [w391]
              stop <- w392 stop-if-true
              n166 = property class="Bus.lvclass"(reference=w395) -> ("Accessors:EventModuleID"=w394:i32)  [unwired: 1 in, 2 out]
              n167 = Equal?(x=w394, y=w393) -> (x = y?=w392:bool)
            }
            n168 = Variant To Data(type=T4 [] ("clEvtReportArray"), Variant=w388) -> (data=w386:T4)  [unwired: 1 in, 1 out]
            n169 = Bundle By Name(cluster=T19 {"BusIndex"=0, "clImpairReportArray"=[]} ("clEvtReportArray"), "BusIndex"=w389, "clImpairReportArray"=w386) -> (w384:T19)
            n170 = local read "QueName"() -> (w380:string)
            n171 = call "Enqueue.vi"("QueName"=w380, "Data"=w384, "Message"="PmuImpairRpt") -> ("Error"=w385:errorcluster[])  [unwired: 8 in]
          }
        }
      }
      event User Event {
        # "Enabled?"
        n172 = event-data() -> ("ModuleID"=w400:i32, "Data"=w399:variant)  [unwired: 1 in]
        n173 = case shown="True" TRUE {
          tunnel: w401 -> [w402 w404]
          tunnel: w400 -> [_ w413]
          tunnel: w399 -> [_ w411]
          tunnel: [_ w408] -> w398
          tunnel: [w402 w404] -> w396
          frame False {
          }
          frame True {
            # "Find Bus Index"
            n174 = for {
              tunnel: w404 -> [w418] mode=indexing
              tunnel: w413 -> [w416]
              tunnel: [w414] -> w412
              i -> [w414]
              stop <- w415 stop-if-true
              n175 = property class="Bus.lvclass"(reference=w418) -> ("Accessors:EventModuleID"=w417:i32)  [unwired: 1 in, 2 out]
              n176 = Equal?(x=w417, y=w416) -> (x = y?=w415:bool)
            }
            n177 = Variant To Data(type=T7 [] ("dblNetworkTime"), Variant=w411) -> (data=w409:T7)  [unwired: 1 in, 1 out]
            n178 = Bundle By Name(cluster=T20 {"BusIndex"=0, "clNetImpairTimeArray"=[]} ("clEvtReportArray"), "BusIndex"=w412, "clNetImpairTimeArray"=w409) -> (w407:T20)
            n179 = local read "QueName"() -> (w403:string)
            n180 = call "Enqueue.vi"("QueName"=w403, "Data"=w407, "Message"="NetImpairTime") -> ("Error"=w408:errorcluster[])  [unwired: 8 in]
          }
        }
      }
      event User Event {
        # "Enabled?"
        n181 = event-data() -> ("ModuleID"=w423:i32, "Data"=w422:variant)  [unwired: 1 in]
        n182 = case shown="True" TRUE {
          tunnel: w424 -> [w425 w427]
          tunnel: w423 -> [_ w436]
          tunnel: w422 -> [_ w434]
          tunnel: [_ w431] -> w421
          tunnel: [w425 w427] -> w419
          frame False {
          }
          frame True {
            # "Find Bus Index"
            n183 = for {
              tunnel: w427 -> [w441] mode=indexing
              tunnel: w436 -> [w439]
              tunnel: [w437] -> w435
              i -> [w437]
              stop <- w438 stop-if-true
              n184 = property class="Bus.lvclass"(reference=w441) -> ("Accessors:EventModuleID"=w440:i32)  [unwired: 1 in, 2 out]
              n185 = Equal?(x=w440, y=w439) -> (x = y?=w438:bool)
            }
            n186 = Variant To Data(type=T8 [] ("dblPktLoss"), Variant=w434) -> (data=w432:T8)  [unwired: 1 in, 1 out]
            n187 = Bundle By Name(cluster=T21 {"BusIndex"=0, "clNetPktLoss"=[]} ("clEvtReportArray"), "BusIndex"=w435, "clNetPktLoss"=w432) -> (w430:T21)
            n188 = local read "QueName"() -> (w426:string)
            n189 = call "Enqueue.vi"("QueName"=w426, "Data"=w430, "Message"="NetPktLoss") -> ("Error"=w431:errorcluster[])  [unwired: 8 in]
          }
        }
      }
      event User Event {
        # "Enabled?"
        n190 = event-data() -> ("ModuleID"=w446:i32, "Data"=w445:variant)  [unwired: 1 in]
        n191 = case shown="True" TRUE {
          tunnel: w447 -> [w448 w450]
          tunnel: w446 -> [_ w459]
          tunnel: w445 -> [_ w457]
          tunnel: [_ w454] -> w444
          tunnel: [w448 w450] -> w442
          frame False {
          }
          frame True {
            # "Find Bus Index"
            n192 = for {
              tunnel: w450 -> [w464] mode=indexing
              tunnel: w459 -> [w462]
              tunnel: [w460] -> w458
              i -> [w460]
              stop <- w461 stop-if-true
              n193 = property class="Bus.lvclass"(reference=w464) -> ("Accessors:EventModuleID"=w463:i32)  [unwired: 1 in, 2 out]
              n194 = Equal?(x=w463, y=w462) -> (x = y?=w461:bool)
            }
            n195 = Variant To Data(type=T9 [] ("ui32FlagImpairmentArray"), Variant=w457) -> (data=w455:T9)  [unwired: 1 in, 1 out]
            n196 = Bundle By Name(cluster=T22 {"BusIndex"=0, "FlagImpairArray"=[]} ("clEvtReportArray"), "BusIndex"=w458, "FlagImpairArray"=w455) -> (w453:T22)
            n197 = local read "QueName"() -> (w449:string)
            n198 = call "Enqueue.vi"("QueName"=w449, "Data"=w453, "Message"="FlagImpair") -> ("Error"=w454:errorcluster[])  [unwired: 8 in]
          }
        }
      }
      event "btnStop": Value Change {
        n199 = event-data() -> ()  [unwired: 1 in, 1 out]
        n200 = call "ObtainRequestEvents.vi"() -> ("Error"=w475:errorcluster[], "clRequestEvents"=w472:T10)  [unwired: 10 in]
        n201 = Unbundle By Name(w472) -> ("StopRequest"=w473:refnum<user-event>)
        n202 = Generate User Event(priority (normal)=usereventprio."high priority", user event=w473, event data cluster=T24 {"BusIndex"=0, "Data"=variant} ("event data")) -> (error out=w474:errorcluster)  [unwired: 1 in, 1 out]
        n203 = call <userlib>:"AddError.vi"("Severity"="Fatal" ("String"), "Priority"=u8 0, "ErrorArray"=w475, "error in (no error)"=w474) -> ("ErrorArray"=w471:errorcluster[], "error out"=w468:errorcluster)  [unwired: 6 in]
        n204 = call <vilib>:"Clear Errors.vi"("error in (no error)"=w468) -> ()  [unwired: 5 in, 2 out]
      }
    }
    n205 = local read "QueName"() -> (w246:string)
    n206 = call "EnqueError.vi"("QueName"=w246, "Error"=w251) -> ("Error"=w250:errorcluster[])  [unwired: 9 in]
  }
  n207 = Build Array (concatenate)(w29, w30) -> (w2:errorcluster[])
  "ErrorArray" <- w2
  n208 = Index Array(array=w2) -> (element=w1:errorcluster)  [unwired: 1 in]
  n209 = invoke class="VI" method="FP.Close"(error in=w1) -> ()  [unwired: 2 in, 3 out]
